vi "Read Unique Identifier.vi"(8 "error in (no error)":errorcluster, 11 "Measurement Done in":refnum<class "Measurement Done.lvclass">) -> (0 "error out":errorcluster, 2 "Unique Identifier":string, 3 "Measurement Done out":refnum<class "Measurement Done.lvclass">)   [LabVIEW 2015, in "Controller Actor.lvlib" / "Measurement Done.lvclass"]
uses:
  Measurement Done.lvclass
  Measurement Done.lvclass/Measurement Done.ctl
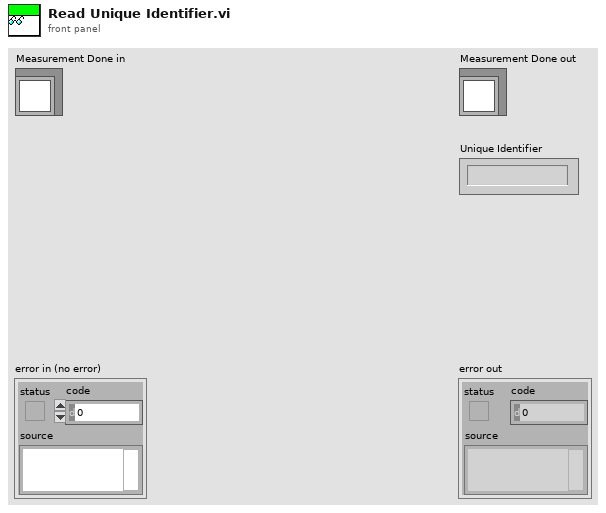
[diagram p1: front panel]
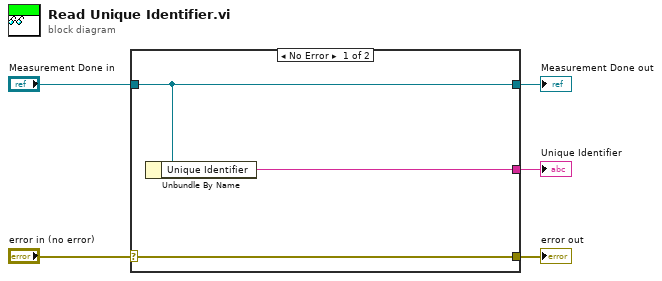
[diagram p0: block diagram]
diagram:
  n1 = case shown="No Error" "error in (no error)" {
    selector: "error in (no error)" -> [w8 w9]
    tunnel: [w8 w9] -> w4
    tunnel: [w7 w10] -> w2
    tunnel: "Measurement Done in" -> [w7 w10]
    tunnel: [w6 _] -> w1
    frame No Error {
      n2 = Unbundle By Name(w7) -> ("Unique Identifier"=w6:string)
    }
    frame Error {
    }
  }
  "error out" <- w4
  "Measurement Done out" <- w2
  "Unique Identifier" <- w1
